vi "vibratome3 module.vi"(7 "Action":T1, 8 "error in":errorcluster) -> (0 "error out":errorcluster)   [LabVIEW 2018]
uses:
  Controls/vibratome3 control.ctl
  Controls/FGV Actions.ctl
  <vilib>/DAQmx/write.llb/DAQmx Write (Analog 1D DBL 1Chan NSamp).vi
  <vilib>/DAQmx/create/channels.llb/DAQmx Create Channel (AO-Voltage-Basic).vi
  <vilib>/DAQmx/configure/timing.llb/DAQmx Timing (Sample Clock).vi
  <vilib>/DAQmx/miscellaneous.llb/DAQmx Fill In Error Info.vi
  <resource>/objmgr/daqmx.rc
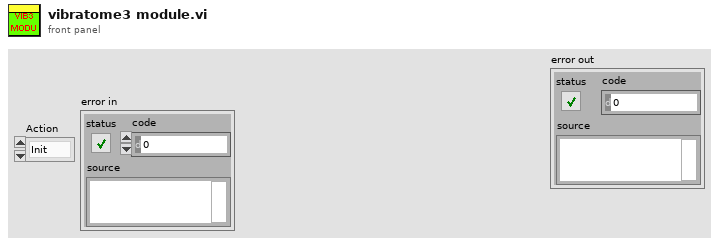
[diagram p1: front panel]
types:
  T1 = typedef "vibratome3 control.ctl" = enum16{"Init", "Configure channel", "Write waveform", "Start", "Stop", "Finish?", "Uninit"}
  T2 = typedef "FGV Actions.ctl" = enum16{"Init", "Set", "Get", "Clear"}
  T3 = typedef "System Parameters.ctl" = cluster{"Optical Parameters":T4, "Vibratome":T5, "Table Stages":T6, "Imaging Parameter":T9, "Galvo HW Parameters":cluster{"Analog Out Channel":tag, "Min Voltage":dbl, "Max Voltage":dbl, "Pixel Clock Source":tag, "Sample Rate":dbl, "Line Clock Out Ch":tag}, "Alazar parameters":T11, "Mosaic Paramter":cluster{"X Axis":cluster{"Start [mm]":dbl, "Steps [pts]":dbl, "End [mm]":dbl}, "Y Axis":cluster{"Start [mm]":dbl, "Steps [pts]":dbl, "End [mm]":dbl}, "Scan Pattern":enum16{"Uni-directional", "Bi-Directional", "Spiral Out", "Spiral In"}, "Overlap Options":cluster{"Overlap Type":enum16{"No Overlap", "X Only", "Y Only", "X and Y"}, "Percent Overlap":u8, "Justify":enum16{"Start", "Center", "End"}}}, "Manual Controls":T18, "Vibratome Axis":T21}
  T4 = typedef "Optical Parameters.ctl" = cluster{"Obj. Focal Length [mm]":dbl, "Scan Lens EFL[mm]":dbl, "Tube Lens EFL[mm]":dbl, "Galvo V Range (+/-)":dbl, "Galvo Max Half Angle [Deg]":dbl, "Max Galvo Range[%]":dbl}
  T5 = typedef "Vibratome Parameters.ctl" = cluster{"Z Bottom [mm]":dbl, "Pre Cut Dwell [s]":dbl, "Blade Frequency [RPM]":u16, "Slice Speed [mm/s]":dbl, "Post Cut Dwell [s]":dbl, "Ramp Time [s]":dbl, "Start X [mm]":dbl, "Start Y [mm]":dbl, "Slice Length [mm]":dbl, "Slice Axis":enum16{"X Axis", "Y Axis", "Z Axis"}, "Controller VISA Ref":refnum<visa-resource-name>, "Blade Frequency [Hz]":u16, "Analog Out Channel":tag, "Pixel Clock Source":tag}
  T6 = typedef "Translation Stage Parameters.ctl" = cluster{"X Stage":T7, "Y Stage":T7, "Z Stage":T7}
  T7 = typedef "Translation Stage Cluster.ctl" = cluster{"Position":dbl, "Is.Enabled?":bool, "Is.Connected?":bool, "Device SN":string, "AccelerationMaximum":dbl, "VelocityMaximum":dbl, "Acceleration":dbl, "Velocity":dbl, "waitTimeout (ms)":i32, "Model":T8, "Is.Homed?":bool, "MOVE":bool}
  T8 = typedef "Translation Stage Types.ctl" = enum16{"None", "Thorlabs LTS", "Thorlabs MLJ"}
  T9 = typedef "Imaging Parameters.ctl" = cluster{"Raster Scan Direction":T10, "Pixel Dwell Time [Clock Cycles]":u16, "Flyback Time [Clock Cycles]":u16, "XY Center [um]":cluster{"X":dbl, "Y":dbl}, "Pixel Step Size [um] X":dbl, "XY Image Size":enum16{"32 x 32", "64 x 64", "128 x 128", "256 x 256", "512 x 512", "1024 x 1024", "2048 x 2048"}, "Custom":bool, "Custom Size":cluster{"X":u16, "Y":u16}, "Line Averages":u8, "Pixel Step Size [um] Y":dbl}
  T10 = typedef "Scan Direction.ctl" = enum16{"Uni Directional", "Bi Directional", "None"}
  T11 = typedef "Alazar parameters.ctl" = cluster{"Trigger Settings":cluster{"General Trigger Settings":T12, "Trigger Engine 1":T13, "Trigger Engine 2":T13}, "Device ID":T14, "Ch A Input Control":T15, "Ch B Input Control":T15, "Acq Settings":T16, "Capture Clock":T17}
  T12 = typedef "General Trigger Settings.ctl" = cluster{"Trigger Operation":u32, "Coupling ID":u32, "Range ID":u32, "Delay":u32, "Timeout Ticks":u32, "Mode":u32, "Parameter":u32}
  T13 = typedef "Trigger Engine Controls.ctl" = cluster{"Trigger Engine":u32, "Source":u32, "Slope":u32, "Level":u32}
  T14 = typedef "Alazar Device ID.ctl" = cluster{"System ID":u32, "Board ID":u32}
  T15 = typedef "Channel Input Controls.ctl" = cluster{"Channel":u8, "Coupling":u32, "Range":u32, "Impedance":u32}
  T16 = typedef "Alazar Acquisition Settings.ctl" = cluster{"Record Length":u32, "Offset":u32, "Records Per Buffer":u32, "Records Count (Records/Acq)":u32, "Window Type":u32, "Footer":u32, "Samples per record":u32, "Output Format":u32}
  T17 = typedef "Clock Controls.ctl" = cluster{"Sample Rate":u32, "Decimation":u32, "Source":u32, "Edge":u32}
  T18 = typedef "Manual Controls.ctl" = cluster{"Z0":dbl, "First image height":dbl, "Data Path":path, "Save parameters":T19, "Center Galvos":bool, "Acquisition mode":T20, "PSOCT Channel":u32, "Save":bool, "AIP rotation angle":dbl, "ret ds":bool, "Pause?":bool, "Outgoing Mail Server (SMTP)":string, "Email":string, "Password":string, "Carrier 1":enum16{"T-Mobile", "AT&T", "Verizon", "Sprint"}, "phone number 1":string, "Subject":string, "Message":string, "blocker position":enum16{"every two slices", "Nat slices", "None"}, "Carrier 2":enum16{"T-Mobile", "AT&T", "Verizon", "Sprint"}, "phone number 2":string}
  T19 = typedef "FFT parameters.ctl" = cluster{"start pixel":i32, "#pixels to save":i32}
  T20 = typedef "FFT mode.ctl" = enum16{"ThorOCT B line", "ThorOCT Spectral", "ThorOCT FFT", "Alazar B line", "Alazar FFT", "GPU FFT", "Alazar Spectral", "Simulation", "auto adjust focus", "Save all"}
  T21 = typedef "Vibratome Param.ctl" = cluster{"Start [mm](first cut height)":dbl, "slice thickness[um]":dbl, "#slice":u16, "image thickness(um)":dbl, "#images":u16, "30um?":bool}
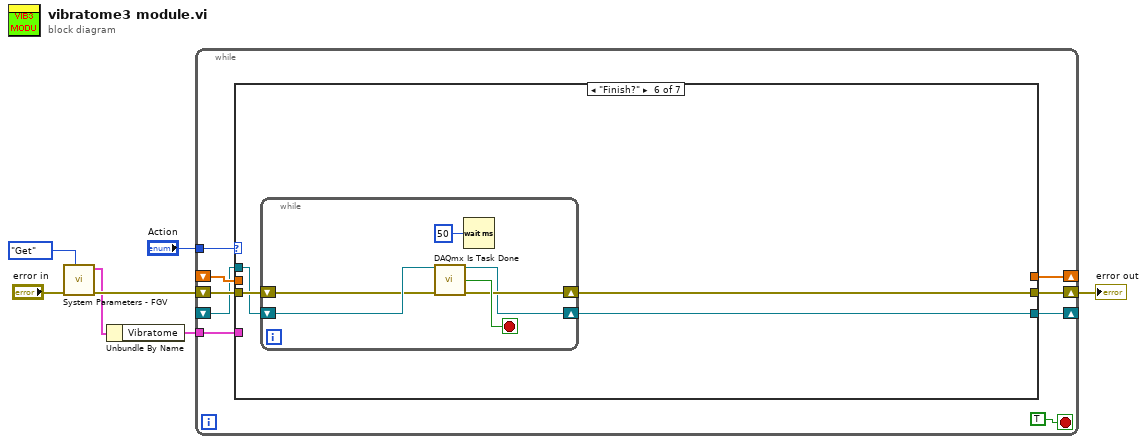
[diagram p0: block diagram]
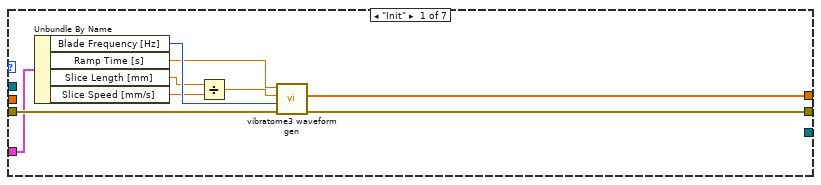
[diagram p2: hidden frame]
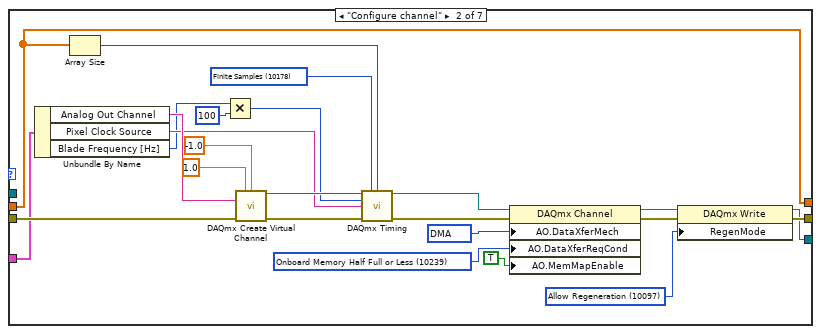
[diagram p3: hidden frame]
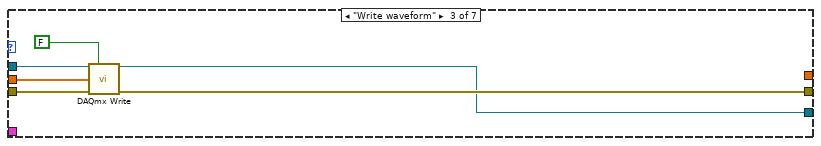
[diagram p4: hidden frame]
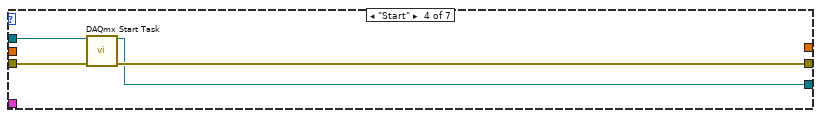
[diagram p5: hidden frame]
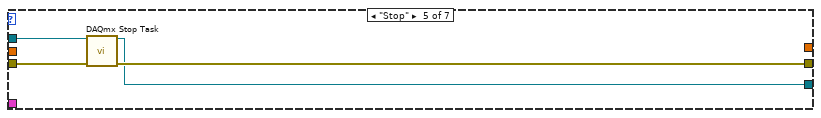
[diagram p6: hidden frame]
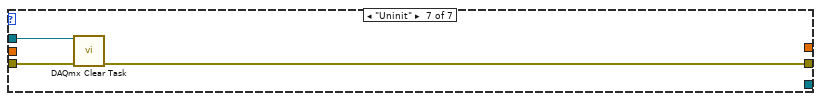
[diagram p7: hidden frame]
diagram:
  n1 = call "System Parameters - FGV.vi"("Actions"=FGV_Actions."Get", "Error In"="error in") -> ("Error Out"=w4:errorcluster, "System Parameters [Out]"=w2:T3)  [unwired: 8 in]
  n2 = Unbundle By Name(w2) -> ("Vibratome"=w1:T5)
  n3 = while {
    tunnel: "Action" -> [w13]
    shift-right: [w15] -> w6
    shift-left: w4 -> [w16]
    shift-right: [w14] -> _
    shift-left: _ -> [w11]
    shift-right: [w12] -> _
    shift-left: _ -> [w10]
    tunnel: w1 -> [w8]
    stop <- TRUE stop-if-true
    n4 = case shown="\"Finish?\"" w13 {
      tunnel: w16 -> [w25 w35 w54 w59 w63 w67 w76]
      tunnel: [w24 w34 w53 w58 w62 w64 w74] -> w15
      tunnel: [w23 w32 _ _ _ _ _] -> w14
      tunnel: [_ w33 w50 w56 w61 w65 _] -> w12
      tunnel: w11 -> [_ w32 w52 _ _ _ _]
      tunnel: w10 -> [_ _ w51 w57 w60 w66 w75]
      tunnel: w8 -> [w22 w31 _ _ _ _ _]
      frame "Init" {
        n5 = Unbundle By Name(w22) -> ("Blade Frequency [Hz]"=w21:u16, "Ramp Time [s]"=w20:dbl, "Slice Length [mm]"=w18:dbl, "Slice Speed [mm/s]"=w17:dbl)
        n6 = Divide(x=w18, y=w17) -> (x/y=w19:dbl)
        n7 = call "vibratome3 waveform gen.vi"("error in"=w25, "frequency(HZ)"=w21, "slice time"=w19, "ramp time(s)"=w20) -> ("error out"=w24:errorcluster, "vib wave"=w23:dbl[])  [unwired: 6 in]
      }
      frame "Configure channel" {
        w46 = 10178 items=["Finite Samples"=10178, "Continuous Samples"=10123, "Hardware Timed Single Point"=12522] ("sample mode")
        w41 = 10097 items=["Allow Regeneration"=10097, "Do Not Allow Regeneration"=10158] ("RegenMode")
        w44 = 10239 items=["Onboard Memory Empty"=10235, "Onboard Memory Half Full or Less"=10239, "Onboard Memory Less than Full"=10242] ("AO.DataXferReqCond")
        w45 = 10054 items=["DMA"=10054, "Interrupts"=10204, "Programmed I/O"=10264, "USB Bulk"=12590] ("AO.DataXferMech")
        n8 = Unbundle By Name(w31) -> ("Analog Out Channel"=w30:tag, "Pixel Clock Source"=w29:tag, "Blade Frequency [Hz]"=w27:u16)
        n9 = Array Size(array=w32) -> (size(s)=w37:i32)
        n10 = Multiply(x=w27, y=u16 100) -> (x*y=w28:u16)
        n11 = call-poly <vilib>:"DAQmx Create Virtual Channel.vi"("maximum value"=1.0, "minimum value"=-1.0, "physical channels"=w30, "error in"=w35) -> ("task out"=w48:refnum<k21>, "error out"=w47:errorcluster)  [unwired: 10 in]
        n12 = call-poly <vilib>:"DAQmx Timing.vi"("task/channels in"=w48, "sample mode"=w46, "samples per channel"=w37, "rate"=w28, "source"=w29, "error in"=w47) -> ("task out"=w38:refnum<k21>, "error out"=w39:errorcluster)  [unwired: 8 in]
        n13 = property class="DAQmx Channel"(reference=w38, error in=w39, "AO.DataXferMech"=w45, "AO.DataXferReqCond"=w44, "AO.MemMapEnable"=TRUE) -> (reference out=w42:refnum<k21>, error out=w36:errorcluster)
        n14 = property class="DAQmx Write"(reference=w42, error in=w36, "RegenMode"=w41) -> (reference out=w33:refnum<k21>, error out=w34:errorcluster)
      }
      frame "Write waveform" {
        n15 = call-poly <vilib>:"DAQmx Write.vi"("task/channels in"=w51, "auto start"=FALSE, "data"=w52, "error in"=w54) -> ("task out"=w50:refnum<k21>, "error out"=w53:errorcluster)  [unwired: 9 in, 1 out]
      }
      frame "Start" {
        n16 = call <vilib>:"DAQmx Start Task.vi"("task/channels in"=w57, "error in"=w59) -> ("task out"=w56:refnum<k21>, "error out"=w58:errorcluster)  [unwired: 12 in]
      }
      frame "Stop" {
        n17 = call <vilib>:"DAQmx Stop Task.vi"("task/channels in"=w60, "error in"=w63) -> ("task out"=w61:refnum<k21>, "error out"=w62:errorcluster)  [unwired: 12 in]
      }
      frame "Finish?" {
        n18 = while {
          shift-right: [w71] -> w65
          shift-left: w66 -> [w70]
          shift-right: [w72] -> w64
          shift-left: w67 -> [w69]
          stop <- w73 stop-if-true
          n19 = call <vilib>:"DAQmx Is Task Done.vi"("task/channels in"=w70, "error in"=w69) -> ("task out"=w71:refnum<k21>, "task done?"=w73:bool, "error out"=w72:errorcluster)  [unwired: 11 in]
          n20 = Wait (ms)(milliseconds to wait=u32 50) -> ()  [unwired: 1 out]
        }
      }
      frame "Uninit" {
        n21 = call <vilib>:"DAQmx Clear Task.vi"("task in"=w75, "error in"=w76) -> ("error out"=w74:errorcluster)  [unwired: 13 in]
      }
    }
  }
  "error out" <- w6
